vi "FGV_bank_account.vi"(7 "Menu":enum16{"Read", "Subtract", "Add"}(ring), 8 "error in (no error)":errorcluster, 11 "input":dbl) -> (0 "error out":errorcluster, 3 "Output":dbl)   [LabVIEW 2022 SP3]
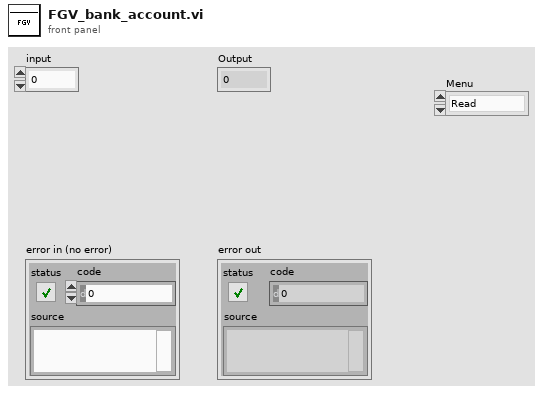
[diagram p1: front panel]
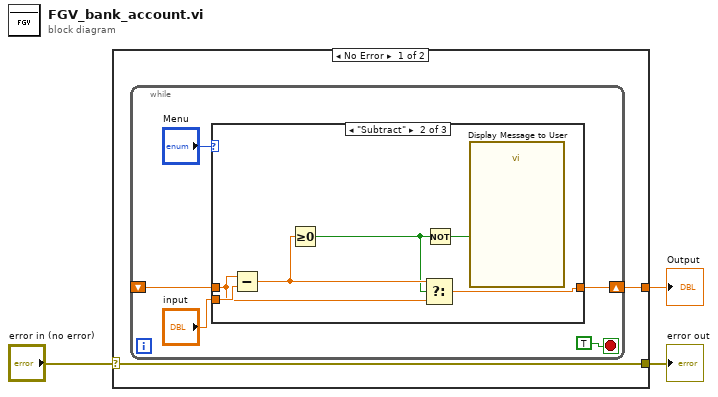
[diagram p0: block diagram]
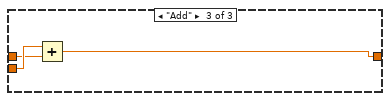
[diagram p3: hidden frame]
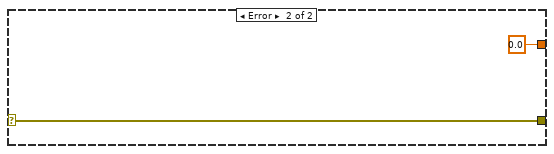
[diagram p4: hidden frame]
diagram:
  n1 = case shown="No Error" "error in (no error)" {
    selector: "error in (no error)" -> [w4 w22]
    tunnel: [w5 0.0] -> w3
    tunnel: [w4 w22] -> w1
    frame No Error {
      n2 = while {
        shift-right: [w10] -> w5
        shift-left: _ -> [w9]
        stop <- TRUE stop-if-true
        n3 = case shown="\"Subtract\"" "Menu" {
          tunnel: [w11 w15 w18] -> w10
          tunnel: w9 -> [w11 w14 w19]
          tunnel: "input" -> [_ w17 w20]
          frame "Read", Default {
          }
          frame "Subtract" {
            n4 = Subtract(x=w14, y=w17) -> (x-y=w16:dbl)
            n5 = Greater Or Equal To 0?(x=w16) -> (x >= 0?=w13:bool)
            n6 = Select(t=w16, s=w13, f=w14) -> (s? t:f=w15:dbl)
            n7 = Not(x=w13) -> (.not. x?=w12:bool)
            n8 = call "Display Message to User"("Enable"=w12) -> ()  [unwired: 9 in, 2 out]
          }
          frame "Add" {
            n9 = Add(x=w20, y=w19) -> (x+y=w18:dbl)
          }
        }
      }
    }
    frame Error {
    }
  }
  "Output" <- w3
  "error out" <- w1
